vi "Get LR700 R & X_VISA.vi"(4 "error in (no error)":errorcluster, 7 "VISA resource name":refnum<visa-resource-name>) -> (0 "error out":errorcluster, 1 "VISA resource name out":refnum<visa-resource-name>, 2 "X":dbl format="%.2e", 3 "Resistance":dbl format="%#_8p")   [LabVIEW 2016]
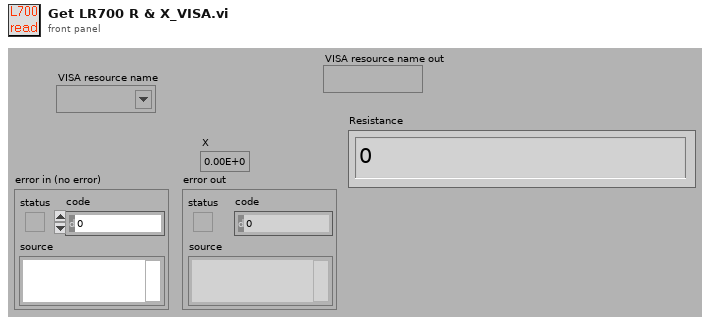
[diagram p1: front panel]
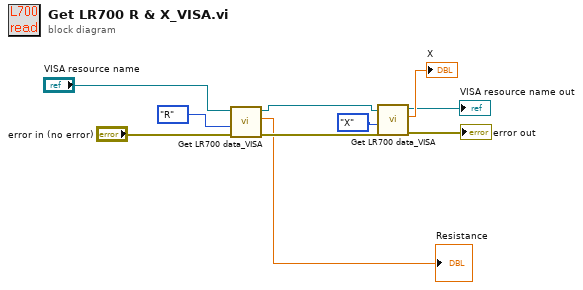
[diagram p0: block diagram]
diagram:
  n1 = call "Get LR700 data_VISA.vi"("error in (no error)"="error in (no error)", "Data chanel"=enum16{"R", "X"}."R", "VISA resource name"="VISA resource name") -> ("error out"=w8:errorcluster, "Data"=→"Resistance":dbl, "VISA resource name out"=w3:refnum<visa-resource-name>)  [unwired: 1 in, 1 out]
  n2 = call "Get LR700 data_VISA.vi"("error in (no error)"=w8, "Data chanel"=enum16{"R", "X"}."X", "VISA resource name"=w3) -> ("error out"=→"error out":errorcluster, "Data"=→"X":dbl, "VISA resource name out"=→"VISA resource name out":refnum<visa-resource-name>)  [unwired: 1 in, 1 out]
